vi "Read Config Parameters.vi"(8 "error in (no error)":errorcluster, 11 "System Modules Factory in":refnum<class "System Modules Factory.lvclass">) -> (0 "error out":errorcluster, 2 "Config Parameters":T1, 3 "System Modules Factory out":refnum<class "System Modules Factory.lvclass">)   [LabVIEW 2024, in "System Modules Factory.lvclass"]
uses:
  System Modules Factory.lvclass
  Type Def/Config Parameters.ctl
  Messenger/Mail Strategy/Mail Strategy.lvclass
  Actor/System Actor/System Actor.lvclass
  System Modules Factory.lvclass/System Modules Factory.ctl
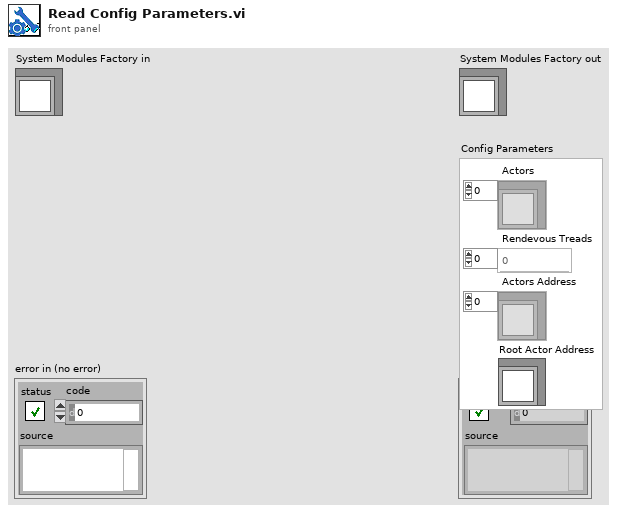
[diagram p1: front panel]
types:
  T1 = typedef "Config Parameters.ctl" = cluster{"Actors":refnum<class "System Actor.lvclass">[], "Rendevous Treads":i32[], "Actors Address":refnum<class "Mail Strategy.lvclass">[], "Root Actor Address":refnum<class "Mail Strategy.lvclass">}
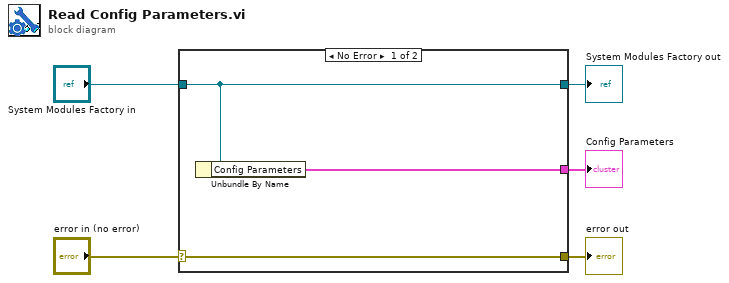
[diagram p0: block diagram]
diagram:
  n1 = case shown="No Error" "error in (no error)" {
    selector: "error in (no error)" -> [w8 w9]
    tunnel: [w8 w9] -> w4
    tunnel: [w7 w10] -> w2
    tunnel: "System Modules Factory in" -> [w7 w10]
    tunnel: [w6 _] -> w1
    frame No Error {
      n2 = Unbundle By Name(w7) -> ("Config Parameters"=w6:T1)
    }
    frame Error {
    }
  }
  "error out" <- w4
  "System Modules Factory out" <- w2
  "Config Parameters" <- w1
